vi "simple_snmp_get.vi"(8 "error in (no error)":errorcluster, 10 "OID Array":string[](array[string]), 11 "IP Address of SNMP Device":string="10.211.1.231") -> (0 "error out":errorcluster, 2 "SnmpDataAsStrings":string[][](array[string]), 4 "SNMP error-status":u8)   [LabVIEW 2017]
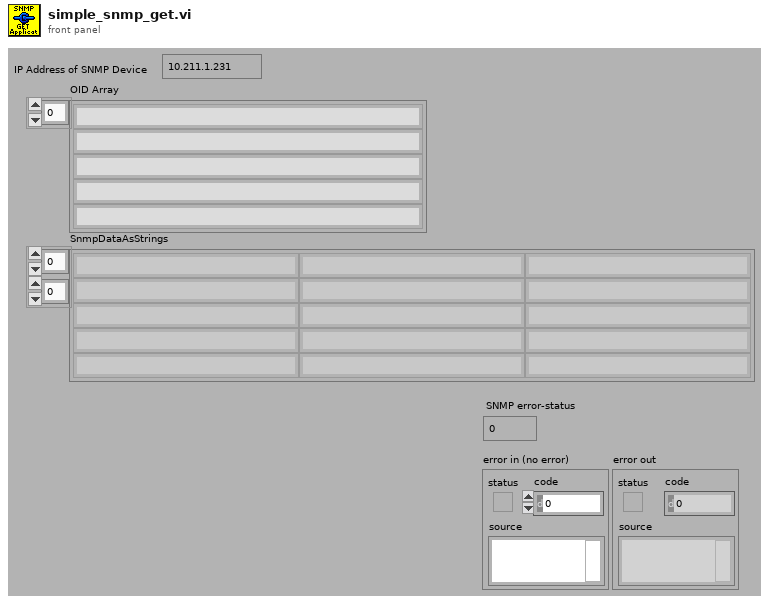
[diagram p1: front panel]
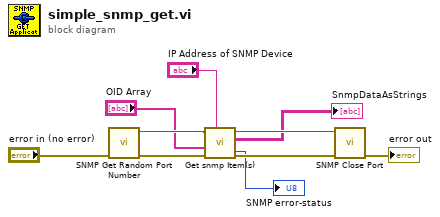
[diagram p0: block diagram]
diagram:
  n1 = call "SNMP Get Random Port Number.vi"("error in (no error)"="error in (no error)") -> ("error out"=w8:errorcluster, "connection ID"=w10:refnum<k16>)  [unwired: 9 out]
  n2 = call "Get snmp Item(s).vi"("IP Address of SNMP Device"="IP Address of SNMP Device", "error in (no error)"=w8, "OID ARRAY"="OID Array", "connection ID in"=w10) -> ("error out"=w7:errorcluster, "SnmpDataAsStrings"=→"SnmpDataAsStrings":string[][], "connection ID out"=w9:refnum<k16>, "error-status"=→"SNMP error-status":u8)  [unwired: 3 in, 1 out]
  n3 = call "SNMP Close Port.vi"("error in (no error)"=w7, "connection ID"=w9) -> ("error out"=→"error out":errorcluster)  [unwired: 9 out]
